vi "DCA Calculate Measurement Values.vi"(1 "Topology":T1, 2 "Measurement Values":T2, 4 "Attenuation Calculation":enum32{"Power", "Voltage"}(ring)) -> (5 "Calculated Measurement Values":T2)   [LabVIEW 2011]
uses:
  TypeDefs/DCA Measurement Values.ctl
  TypeDefs/DCA Topology.ctl
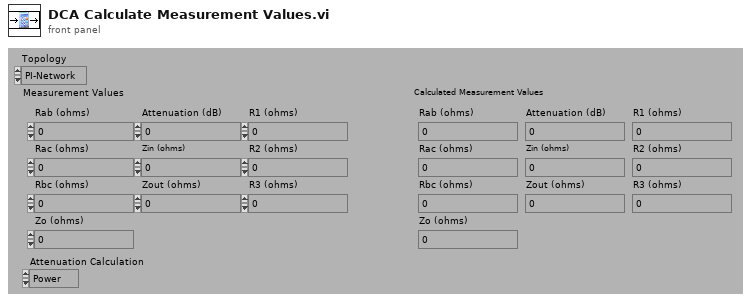
[diagram p1: front panel]
types:
  T1 = typedef "DCA Topology.ctl" = enum32{"PI-Network", "T-Network"}
  T2 = typedef "DCA Measurement Values.ctl" = cluster{"Rab (ohms)":dbl, "Rac (ohms)":dbl, "Rbc (ohms)":dbl, "Zo (ohms)":dbl, "Attenuation (dB)":dbl, "Zin (ohms)":dbl, "Zout (ohms)":dbl, "R1 (ohms)":dbl, "R2 (ohms)":dbl, "R3 (ohms)":dbl}
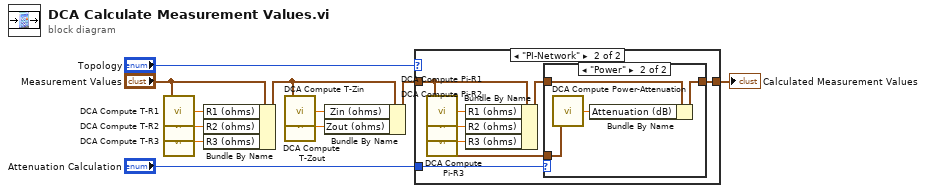
[diagram p0: block diagram]
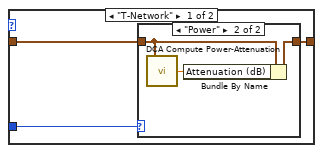
[diagram p2: hidden frame]
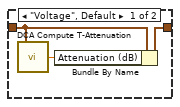
[diagram p3: hidden frame]
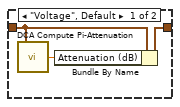
[diagram p4: hidden frame]
diagram:
  n1 = call "DCA Compute T-R1.vi"("Measurement Values"="Measurement Values") -> ("T-R1"=w8:dbl)
  n2 = call "DCA Compute T-R2.vi"("Measurement Values"="Measurement Values") -> ("T-R2"=w10:dbl)
  n3 = call "DCA Compute T-R3.vi"("Measurement Values"="Measurement Values") -> ("T-R3"=w9:dbl)
  n4 = Bundle By Name(cluster="Measurement Values", "R1 (ohms)"=w8, "R2 (ohms)"=w10, "R3 (ohms)"=w9) -> (w2:T2)
  n5 = call "DCA Compute T-Zin.vi"("Measurement Values"=w2) -> ("T-Zin"=w4:dbl)
  n6 = call "DCA Compute T-Zout.vi"("Measurement Values"=w2) -> ("T-Zout"=w3:dbl)
  n7 = Bundle By Name(cluster=w2, "Zin (ohms)"=w4, "Zout (ohms)"=w3) -> (w1:T2)
  n8 = case shown="\"PI-Network\"" "Topology" {
    tunnel: w1 -> [w12 w21]
    tunnel: [w14 w23] -> w11
    tunnel: "Attenuation Calculation" -> [w13 w24]
    frame "T-Network" {
      n9 = case shown="\"Power\"" w13 {
        tunnel: w12 -> [w16 w19]
        tunnel: [w15 w18] -> w14
        frame "Voltage", Default {
          n10 = call "DCA Compute T-Attenuation.vi"("Measurement Values"=w16) -> ("T-Attenuation"=w17:dbl)
          n11 = Bundle By Name(cluster=w16, "Attenuation (dB)"=w17) -> (w15:T2)
        }
        frame "Power" {
          n12 = call "DCA Compute Power-Attenuation.vi"("Measurement Values"=w19) -> ("Power-Attenuation"=w20:dbl)
          n13 = Bundle By Name(cluster=w19, "Attenuation (dB)"=w20) -> (w18:T2)
        }
      }
    }
    frame "PI-Network" {
      n14 = call "DCA Compute Pi-R1.vi"("Measurement Values"=w21) -> ("Pi-R1"=w27:dbl)
      n15 = call "DCA Compute Pi-R2.vi"("Measurement Values"=w21) -> ("Pi-R2"=w26:dbl)
      n16 = call "DCA Compute Pi-R3.vi"("Measurement Values"=w21) -> ("Pi-R3"=w25:dbl)
      n17 = Bundle By Name(cluster=w21, "R1 (ohms)"=w27, "R2 (ohms)"=w26, "R3 (ohms)"=w25) -> (w22:T2)
      n18 = case shown="\"Power\"" w24 {
        tunnel: w22 -> [w29 w33]
        tunnel: [w28 w32] -> w23
        tunnel: w21 -> [_ w31]
        frame "Voltage", Default {
          n19 = call "DCA Compute Pi-Attenuation.vi"("Measurement Values"=w29) -> ("Pi-Attenuation"=w30:dbl)
          n20 = Bundle By Name(cluster=w29, "Attenuation (dB)"=w30) -> (w28:T2)
        }
        frame "Power" {
          n21 = call "DCA Compute Power-Attenuation.vi"("Measurement Values"=w31) -> ("Power-Attenuation"=w34:dbl)
          n22 = Bundle By Name(cluster=w33, "Attenuation (dB)"=w34) -> (w32:T2)
        }
      }
    }
  }
  "Calculated Measurement Values" <- w11
